vi "dfd_Render Coefficients of Difference Equation.vi"(4 "first non-zero coefficient":bool, 5 "[user-specified font]":T3={"Font Name:"="", "Size"=12, "Strikeout?"=FALSE, "Italic?"=FALSE, "Underline?"=FALSE, "Outline?"=FALSE, "Shadow?"=FALSE, "Bold?"=FALSE}, 6 "alignment(left, top)":T2, 7 "format string":string="%#.4g", 9 "rect in":T1, 10 "coefficient":dbl, 11 "picture in":picture) -> (1 "rect out":T1, 3 "picture out":picture)   [LabVIEW 2017, in "NI_DigFilter_Process.lvlib"]
uses:
  <vilib>/addons/Digital Filter Design/NI_DigFilter_Process.lvlib
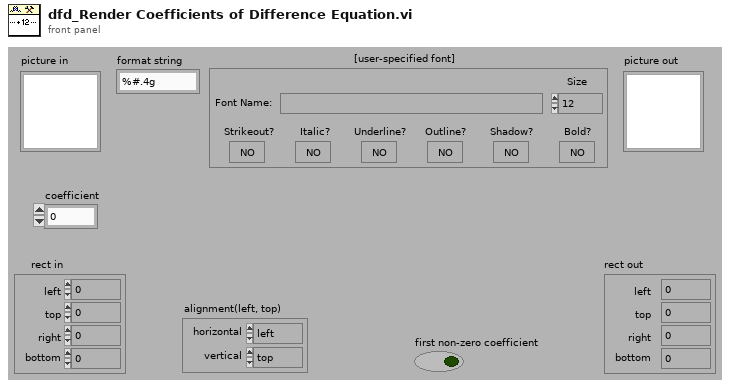
[diagram p1: front panel]
types:
  T1 = cluster{"left":i16, "top":i16, "right":i16, "bottom":i16}
  T2 = cluster{"horizontal":enum16{"left", "center", "right"}, "vertical":enum16{"top", "center", "bottom"}}
  T3 = cluster{"Font Name:":string, "Size":i16, "Strikeout?":bool, "Italic?":bool, "Underline?":bool, "Outline?":bool, "Shadow?":bool, "Bold?":bool}
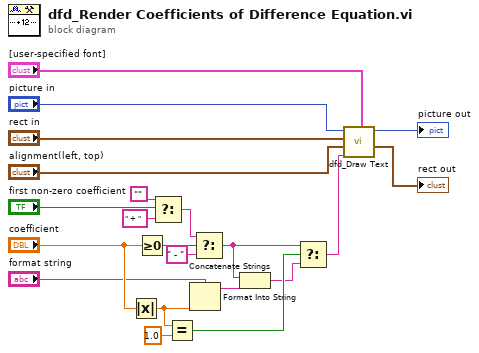
[diagram p0: block diagram]
diagram:
  n1 = Absolute Value(x="coefficient") -> (abs(x)=w6:dbl)
  n2 = Greater Or Equal To 0?(x="coefficient") -> (x >= 0?=w18:bool)
  n3 = Select(t="", s="first non-zero coefficient", f=" + " ("resulting string")) -> (s? t:f=w4:string)
  n4 = Equal?(x=w6, y=1.0) -> (x = y?=w21:bool)
  n5 = Format Into String(format string="format string", w6) -> (resulting string=w17:string)  [unwired: 2 in, 1 out]
  n6 = Select(t=w4, s=w18, f=" - " ("resulting string")) -> (s? t:f=w5:string)
  n7 = Concatenate Strings(w5, w17) -> (w16:string)
  n8 = Select(t=w5, s=w21, f=w16) -> (s? t:f=w12:string)
  n9 = call <vilib>:"dfd_Draw Text.vi"("font input"="[user-specified font]", "text"=w12, "alignment(left, top)"="alignment(left, top)", "rect in"="rect in", "picture in"="picture in") -> ("rect out"=→"rect out":T1, "picture out"=→"picture out":picture)  [unwired: 3 in, 2 out]
